vi "Settings_SubVI.vi"(11 "Main Data Cluster in":T1 {"task ID" format="%.0x"}) -> (3 "Main Data Cluster out":T1 {"task ID" format="%.0x"})   [LabVIEW 2019]
doc: "This SubVI updates Main Data Cluster with the info that the user provided. When \"INFO\" button is clicked github page for the project is opened.\n\nIN: Main Data Cluster in;\nOUT: Main Data Cluster out;"
uses:
  <vilib>/Platform/browser.llb/Open URL in Default Browser (string).vi
  controls/#typedef_Waveform_Type.ctl
  <vilib>/sound2/lvsound2.llb/Sound Data Format.ctl
  <vilib>/sound2/lvsound2.llb/Sound Output Task ID.ctl
  controls/#typedef_Data_Cluster.ctl
panel:
  in  "Sample Rate":dbl
  in  "Device ID":u32
  in  "Help Button":bool
  in  "OK Button":bool
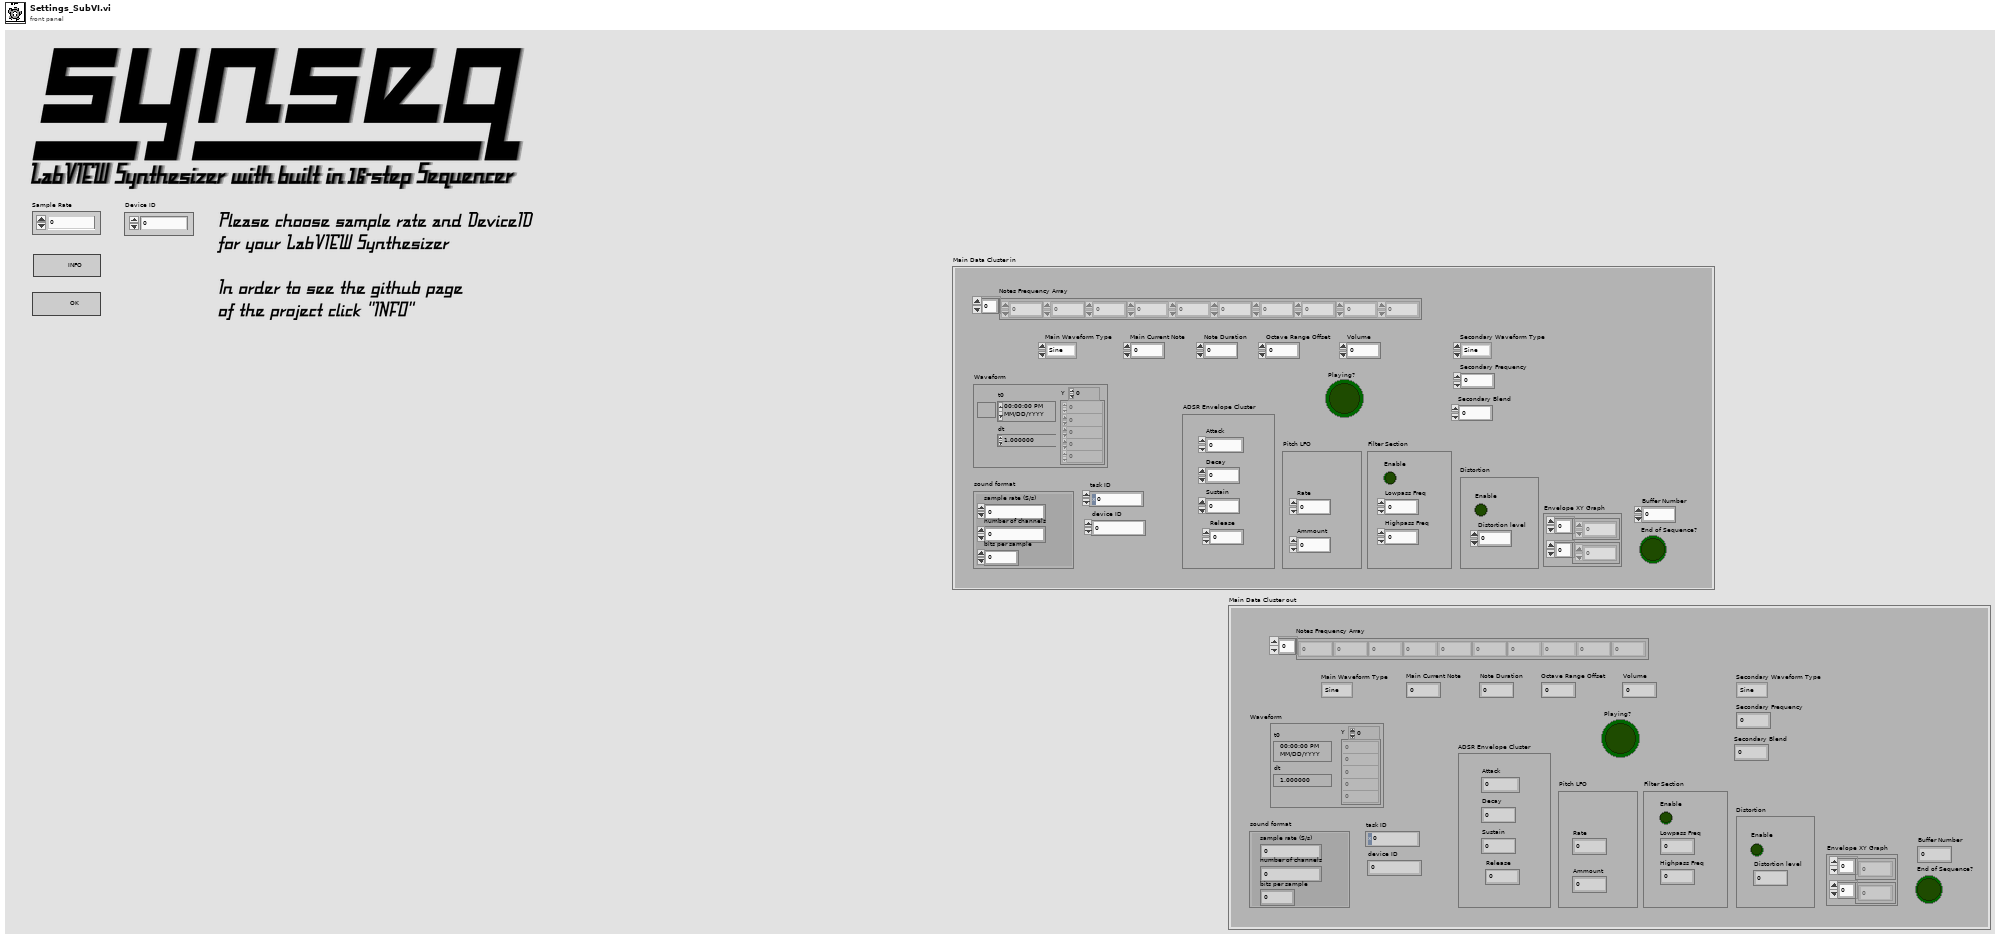
[diagram p1: front panel]
types:
  T1 = typedef "#typedef_Data_Cluster.ctl" = cluster{"Notes Frequency Array":dbl[], "Main Waveform Type":T2, "Waveform":waveform(dbl), "Main Current Note":i32, "Octave Range Offset":u32, "sound format":T3, "Task ID":T4, "Note Duration":dbl, "Volume":dbl, "ADSR Envelope Cluster":cluster{"Decay":i32, "Sustain":i32, "Attack":i32, "Release":i32}, "Playing?":bool, "Pitch LFO":cluster{"Rate":dbl, "Ammount":dbl}, "device ID":u32, "Filter Section":cluster{"Lowpass Freq":dbl, "Highpass Freq":dbl, "Enable":bool}, "Distortion":cluster{"Distortion level":dbl, "Enable":bool}, "Secondary Waveform Type":T2, "Secondary Frequency":dbl, "Secondary Blend":dbl, "Envelope XY Graph":cluster{dbl[], dbl[]}, "Buffer Number":i32, "End of Sequence?":bool}
  T2 = typedef "#typedef_Waveform_Type.ctl" = enum16{"Sine", "Saw", "Square", "Triangle", "Noise"}
  T3 = typedef "Sound Data Format.ctl" = cluster{"sample rate (S/s)":dbl, "number of channels":i32, "bits per sample":i32}
  T4 = typedef "Sound Output Task ID.ctl" = u32
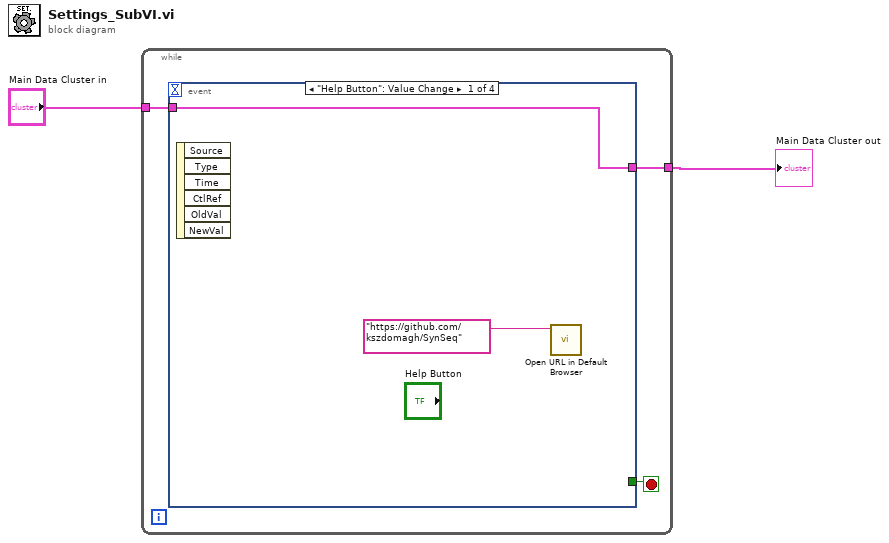
[diagram p0: block diagram]
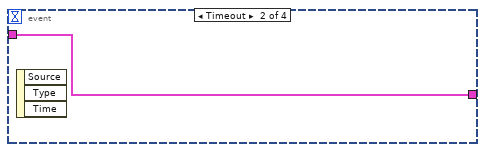
[diagram p2: hidden frame]
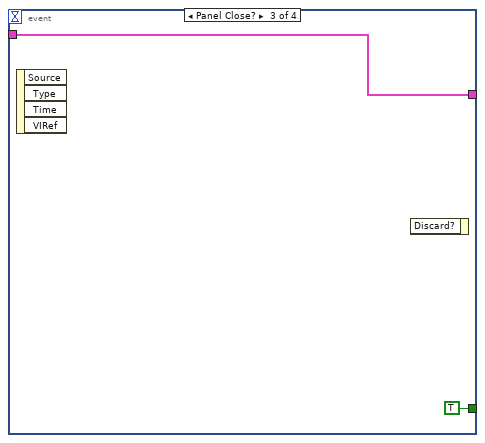
[diagram p3: hidden frame]
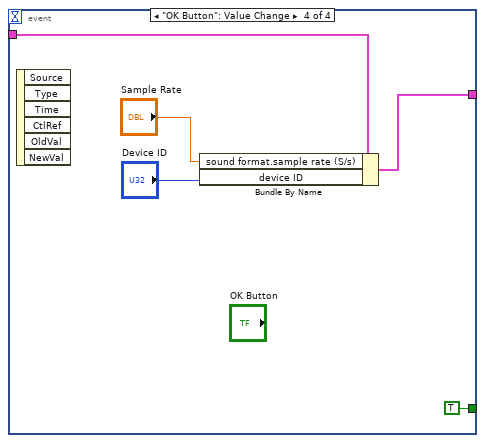
[diagram p4: hidden frame]
diagram:
  n1 = while {
    tunnel: "Main Data Cluster in" -> [w5]
    tunnel: [w3] -> w1
    stop <- w4 stop-if-true
    n2 = event shown="[0] \"Help Button\": Value Change" {
      selector: _ -> [_ _ _ _]
      dyn-events: _ -> [_ _ _ _]
      timeout: _ -> [_ _ _ _]
      tunnel: w5 -> [w7 w8 w9 w13]
      tunnel: [_ _ TRUE ("OK Button") TRUE ("OK Button")] -> w4
      tunnel: [w7 w8 w9 w12] -> w3
      event "Help Button": Value Change {
        n3 = event-data() -> ()  [unwired: 1 in, 6 out]
        n4 = call-poly <vilib>:"Open URL in Default Browser.vi"("URL"="https://github.com/kszdomagh/SynSeq") -> ()  [unwired: 5 in, 2 out]
      }
      event Timeout {
        n5 = event-data() -> ()  [unwired: 1 in, 3 out]
      }
      event Panel Close? {
        n6 = event-data() -> ()  [unwired: 1 in, 4 out]
        n7 = event-data() -> ()  [unwired: 2 in, 1 out]
      }
      event "OK Button": Value Change {
        n8 = event-data() -> ()  [unwired: 1 in, 6 out]
        n9 = Bundle By Name(cluster=w13, "sound format.sample rate (S/s)"="Sample Rate", "device ID"="Device ID") -> (w12:T1)
      }
    }
  }
  "Main Data Cluster out" <- w1
